vi "Color Fix.vi"(0 "Reference Cluster":T1) -> ()   [LabVIEW 2017, in "GUI.lvlib"]
uses:
  GUI.lvlib
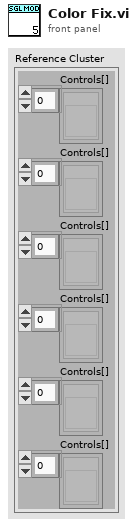
[diagram p1: front panel]
types:
  T1 = cluster{"Controls[]":refnum<vi>[], "Controls[]":refnum<vi>[], "Controls[]":refnum<vi>[], "Controls[]":refnum<vi>[], "Controls[]":refnum<vi>[], "Controls[]":refnum<vi>[]}
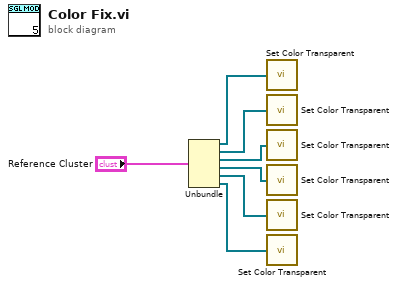
[diagram p0: block diagram]
diagram:
  n1 = Unbundle("Reference Cluster") -> ("Controls[]"=w6:refnum<vi>[], "Controls[]"=w5:refnum<vi>[], "Controls[]"=w4:refnum<vi>[], "Controls[]"=w1:refnum<vi>[], "Controls[]"=w2:refnum<vi>[], "Controls[]"=w3:refnum<vi>[])
  n2 = call "Set Color Transparent.vi"("Controls[]"=w6) -> ()
  n3 = call "Set Color Transparent.vi"("Controls[]"=w5) -> ()
  n4 = call "Set Color Transparent.vi"("Controls[]"=w4) -> ()
  n5 = call "Set Color Transparent.vi"("Controls[]"=w1) -> ()
  n6 = call "Set Color Transparent.vi"("Controls[]"=w2) -> ()
  n7 = call "Set Color Transparent.vi"("Controls[]"=w3) -> ()
